vi "Noise Issues.vi"() -> ()   [LabVIEW 2013]
uses:
  <vilib>/Utility/file.llb/Read From Spreadsheet File (DBL).vi
panel:
  out "Waveform Graph":dbl[][](graph)
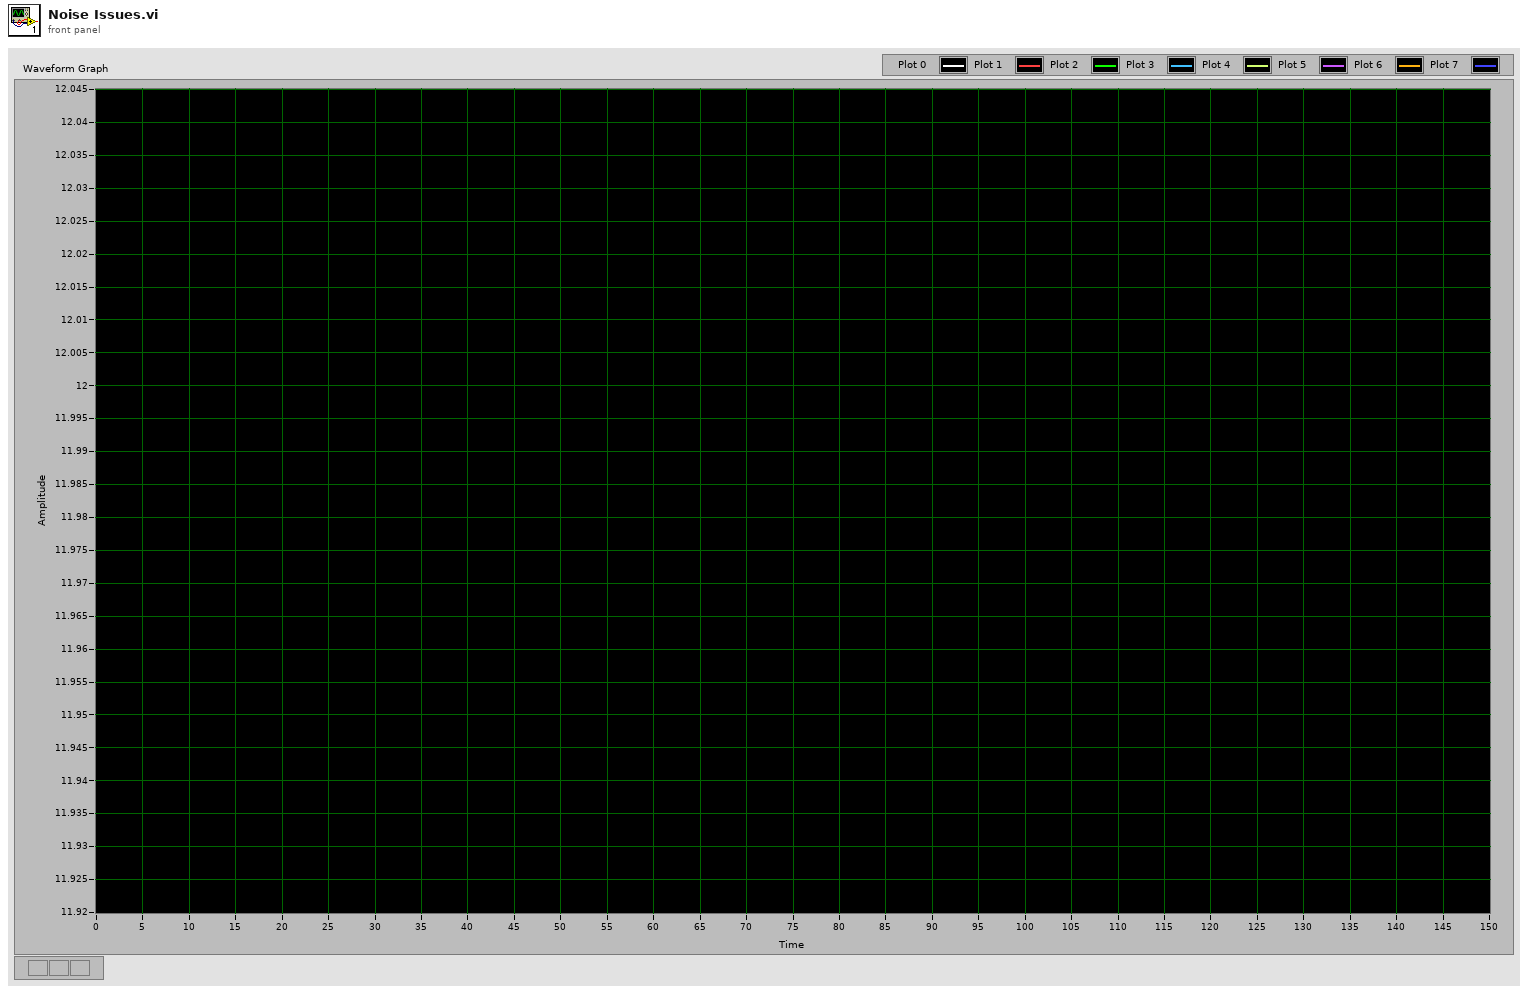
[diagram p1: front panel]
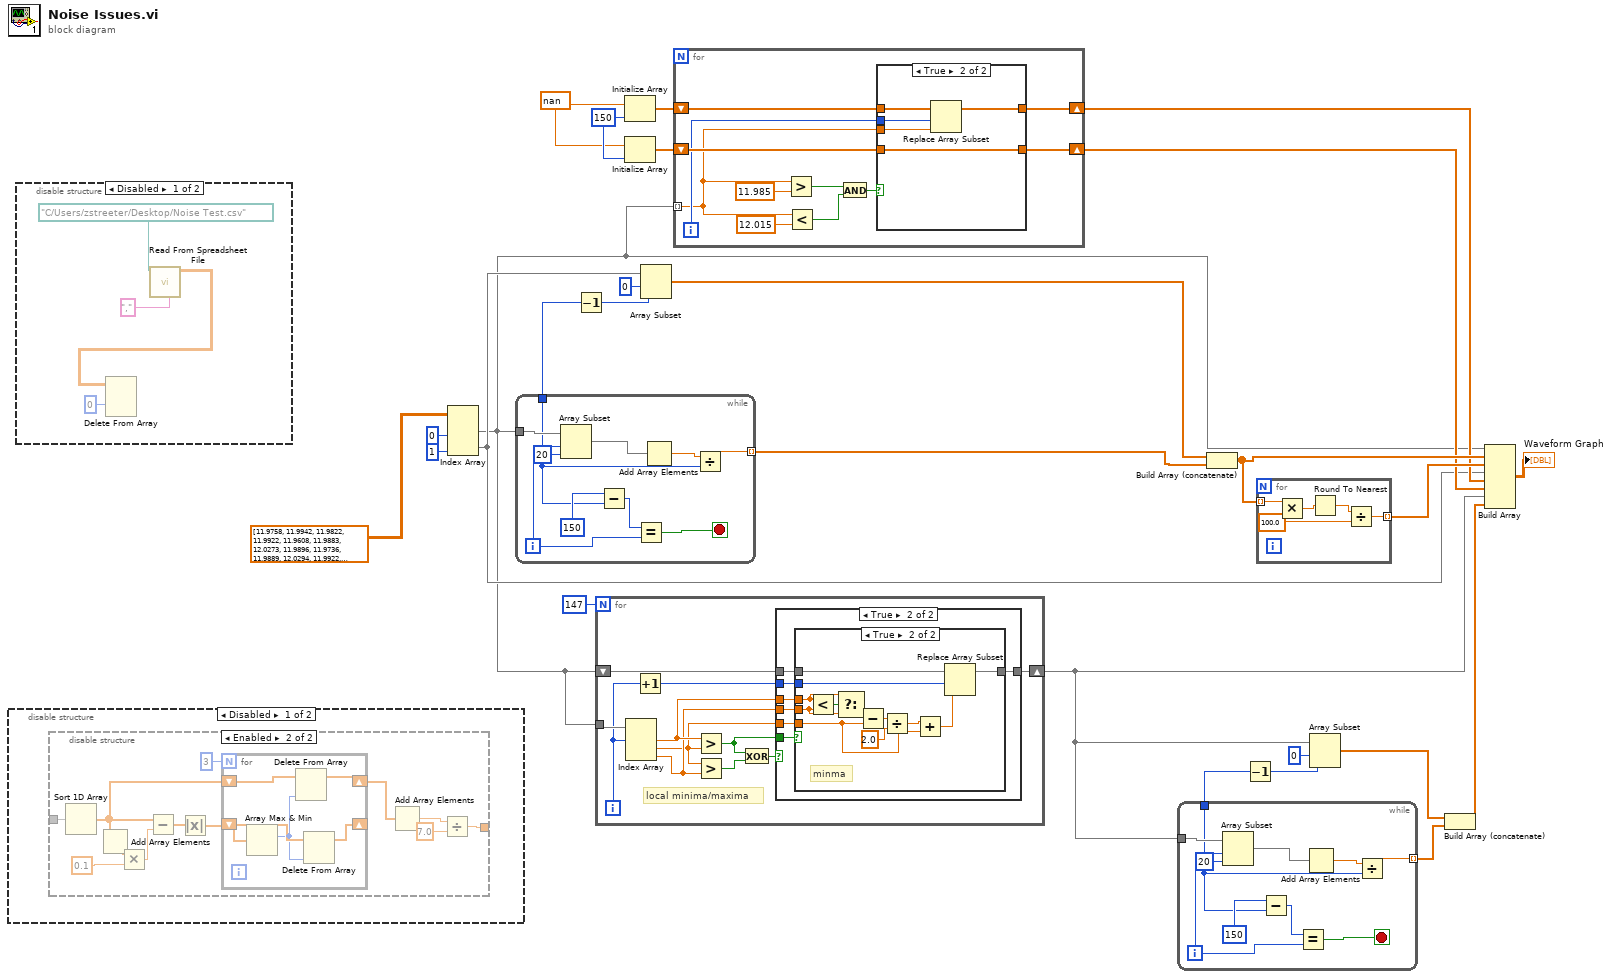
[diagram p0: block diagram]
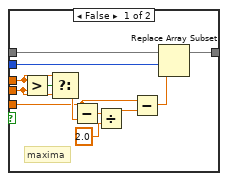
[diagram p3: hidden frame]
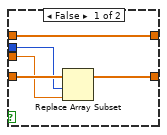
[diagram p4: hidden frame]
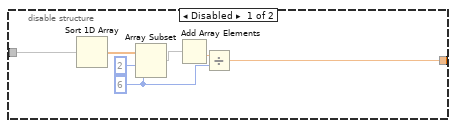
[diagram p6: hidden frame]
diagram:
  w15 = nan
  w16 = 150 ("dimension size")
  n1 = disable-structure shown="Disabled" {
    frame Disabled {
      n2 = disable-structure shown="Enabled" {
        disable-tunnel: _ -> [w34 w46]
        disable-tunnel: [w28 w38] -> _
        frame Disabled {
          w29 = 6 ("length")
          n3 = Sort 1D Array(array=w34) -> (sorted array=w33:ext[])
          n4 = Array Subset(array=w33, index=2, length=w29) -> (w31:ext[])
          n5 = Add Array Elements(numeric array=w31) -> (sum=w30:ext)
          n6 = Divide(x=w30, y=w29) -> (x/y=w28:ext)
        }
        frame Enabled {
          n7 = Sort 1D Array(array=w46) -> (sorted array=w37:ext[])
          n8 = Add Array Elements(numeric array=w37) -> (sum=w44:ext)
          n9 = Multiply(x=w44, y=0.1) -> (x*y=w43:ext)
          n10 = Subtract(x=w37, y=w43) -> (x-y=w41:ext[])
          n11 = Absolute Value(x=w41) -> (abs(x)=w36:ext[])
          n12 = for {
            N: 3 -> [_]
            shift-right: [w50] -> _
            shift-left: w36 -> [w51]
            shift-right: [w48] -> w35
            shift-left: w37 -> [w49]
            n13 = Array Max & Min(array=w51) -> (max index (indices)=w47:i32)  [unwired: 3 out]
            n14 = Delete From Array(array=w49, index=w47) -> (array with subset deleted=w48:ext[])  [unwired: 1 in, 1 out]
            n15 = Delete From Array(array=w51, index=w47) -> (array with subset deleted=w50:ext[])  [unwired: 1 in, 1 out]
          }
          n16 = Add Array Elements(numeric array=w35) -> (sum=w40:ext)
          n17 = Divide(x=w40, y=7.0) -> (x/y=w38:ext)
        }
      }
    }
    frame Enabled {
    }
  }
  n18 = disable-structure shown="Disabled" {
    frame Disabled {
      n19 = call-poly <vilib>:"Read From Spreadsheet File.vi"("delimiter (\\t)"="," ("delimiter (\\t)"), "file path (dialog if empty)"=path "C:/Users/zstreeter/Desktop/Noise Test.csv" ("new file path (Not A Path if cancelled)")) -> ("all rows"=w53:dbl[][])  [unwired: 5 in, 4 out]
      n20 = Delete From Array(array=w53, index (row)=0) -> ()  [unwired: 2 in, 2 out]
    }
    frame Enabled {
    }
  }
  n21 = Index Array(array=dbl[][] [[11.9758, 11.9942], [11.9822, 11.9922], [11.9608, 11.9883], [12.0273, 11.9896], [11.9736, 11.9889], [12.0294, 11.9922], [12.0004, 11.9922], [11.9929, 12.0003], [12.0401, 12.0018], [12.0487, 12.0031], [11.9414, 11.9997], [12.0294, 12.0044], [11.9468, 12.003], [11.8975, 11.99], [11.9811, 11.9908], [11.9543, 11.9833], [11.9715, 11.9804], [12.0358, 11.9847], [11.9511, 11.9758], [12.0101, 11.9719], [11.9736, 11.9751], [11.9779, 11.97], [12.0702, 11.9823], [11.9479, 11.9874], [11.9876, 11.988], [12.0412, 11.9967], [11.9672, 11.9963], [11.9447, 11.9871], [11.9425, 11.9863], [11.9994, 11.9852], [11.9715, 11.985], [11.9726, 11.9845], [12.0326, 11.9807], [11.9575, 11.9817], [12.0176, 11.9847], [11.9264, 11.9732], [12.0165, 11.9781], [11.9468, 11.9783], [11.9962, 11.9837], [12.0627, 11.99], [12.0519, 11.9981], [11.9565, 11.9965], [12.009, 11.9941], [11.9672, 11.9951], [11.9329, 11.9866], [12.0283, 11.9968], [11.9736, 11.9925], [11.9597, 11.9938], [12.0262, 11.9968], [12.0208, 11.9926], [12.0273, 11.9901], [11.9339, 11.9879], [12.0358, 11.9906], [11.9436, 11.9882], [11.964, 11.9913], [12.0326, 11.9918], [11.994, 11.9938], [11.9436, 11.9922], [12.0155, 11.9911], [12.0305, 11.9921], [11.9618, 11.9855], [12.0358, 11.9957], [12.0122, 11.9934], [12.0305, 12.0021], [11.9597, 12.0016], [11.9436, 11.9927], [11.9822, 11.9915], [11.9779, 11.995], [11.9189, 11.9853], [11.9479, 11.9771], [11.9597, 11.9768], [12.0122, 11.9745], [12.0208, 11.9753], [11.9146, 11.9638], [12.0069, 11.9685], [12.0616, 11.9803], [12.0573, 11.9878], [12.0273, 11.9927], [11.9779, 11.9986], [11.9232, 11.9962], [12.067, 12.0069], [11.9532, 12.001], [11.9758, 11.9965], [12.0026, 12.0053], [11.9758, 12.0022], [12.0283, 11.9988], [12.023, 11.9954], [12.0112, 11.9938], [11.9447, 11.9905], [12.0283, 12.001], [11.9726, 11.9915], [11.9833, 11.9945], [12.0176, 11.9987], [12.0305, 12.0015], [12.0358, 12.0075], [12.0358, 12.0083], [11.906, 11.9966], [12.0358, 11.999], [12.0466, 12.0092], [11.9339, 11.9998], [12.0391, 12.0065], [11.9779, 12.0059], [12.0476, 12.0089], [11.9833, 12.0042], [11.9608, 11.9967], [11.9618, 11.9893], [12.0316, 12.0018], [11.9436, 11.9926], [11.964, 11.9844], [12.0112, 11.9921], [12.067, 11.9949], [12.0112, 11.9982], [12.0058, 11.994], [12.067, 12.0024], [12.0584, 12.0121], [11.9586, 12.0118], [11.9243, 12.0011], [12.0273, 12.0095], [11.9361, 12.0067], [12.038, 12.0093], [11.9565, 11.9983], [12.0069, 11.9979], [12.0198, 11.9993], [11.9822, 11.9908], [12.024, 11.9874], [11.9522, 11.9867], [12.038, 11.9981], [11.9693, 11.9923], [12.0251, 12.0012], [11.9726, 11.9947], [11.9972, 11.9987], [12.0423, 12.0023], [12.008, 12.0011], [12.008, 12.0037], [11.9779, 11.999], [12.0208, 12.0059], [11.964, 11.9985], [12.0519, 12.0068], [11.9972, 12.004], [12.0273, 12.0095], [11.9683, 12.0066], [11.9962, 12.0019], [11.9683, 11.998], [11.9962, 11.9968], [12.0594, 12.0049], [11.9726, 12.0001], [12.0466, 12.0084], [12.0112, 12.0043], [11.8953, 11.9941], [12.0219, 11.9936]] ("array w/ subset deleted"), index (col) #1=0 ("disabled index (col)"), index (col) #2=1 ("index (col)")) -> (element #1=w8:dbl[], element #2=w9:dbl[])  [unwired: 2 in]
  n22 = while {
    tunnel: w8 -> [w64]
    tunnel: [w57] -> w19 mode=indexing
    tunnel: [w56] -> w22
    i -> [w63]
    stop <- w62 stop-if-true
    w56 = 20 ("length")
    n23 = Array Subset(array=w64, index=w63, length=w56) -> (w59:dbl[])
    n24 = Subtract(x=150, y=w56) -> (x-y=w60:i32)
    n25 = Equal?(x=w60, y=w63) -> (x = y?=w62:bool)
    n26 = Add Array Elements(numeric array=w59) -> (sum=w58:dbl)
    n27 = Divide(x=w58, y=w56) -> (x/y=w57:dbl)
  }
  n28 = Decrement(x=w22) -> (x-1=w21:i32)
  n29 = for {
    N: 147 -> [_]
    tunnel: w8 -> [w75]
    shift-right: [w71] -> w4
    shift-left: w8 -> [w73]
    i -> [w66]
    # "local minima/maxima"
    n30 = Index Array(array=w75, index #1=w66) -> (element #1=w69:dbl, element #2=w67:dbl, element #3=w68:dbl)  [unwired: 2 in]
    n31 = Increment(x=w66) -> (x+1=w65:i32)
    n32 = Greater?(x=w69, y=w67) -> (0:w70:bool)
    n33 = Greater?(x=w67, y=w68) -> (0:w74:bool)
    n34 = Exclusive Or(1:w74, 2:w70) -> (0:w72:bool)
    n35 = case shown="True" w72 {
      tunnel: w73 -> [w76 w82]
      tunnel: [w76 w78] -> w71
      tunnel: w70 -> [_ w83]
      tunnel: w69 -> [_ w81]
      tunnel: w68 -> [_ w80]
      tunnel: w67 -> [_ w79]
      tunnel: w65 -> [_ w77]
      frame False {
      }
      frame True {
        n36 = case shown="True" w83 {
          tunnel: w82 -> [w87 w103]
          tunnel: w81 -> [w94 w106]
          tunnel: w80 -> [w93 w105]
          tunnel: w79 -> [w89 w96]
          tunnel: [w86 w102] -> w78
          tunnel: w77 -> [w84 w101]
          frame False {
            # "maxima"
            n37 = Greater?(x=w94, y=w93) -> (0:w95:bool)
            n38 = Select(t=w94, s=w95, f=w93) -> (s? t:f=w92:dbl)
            n39 = Subtract(x=w89, y=w92) -> (x-y=w91:dbl)
            n40 = Divide(x=w91, y=2.0) -> (x/y=w88:dbl)
            n41 = Subtract(x=w89, y=w88) -> (x-y=w85:dbl)
            n42 = Replace Array Subset(array=w87, new element=w85, index=w84) -> (w86:dbl[])
          }
          frame True {
            # "minma"
            n43 = Less?(x=w106, y=w105) -> (x < y?=w107:bool)
            n44 = Select(t=w106, s=w107, f=w105) -> (s? t:f=w100:dbl)
            n45 = Subtract(x=w100, y=w96) -> (x-y=w99:dbl)
            n46 = Divide(x=w99, y=2.0) -> (x/y=w98:dbl)
            n47 = Add(x=w98, y=w96) -> (x+y=w97:dbl)
            n48 = Replace Array Subset(array=w103, new element=w97, index=w101) -> (w102:dbl[])
          }
        }
      }
    }
  }
  n49 = Initialize Array(w15, w16) -> (w14:dbl[])
  n50 = Initialize Array(w15, w16) -> (w13:dbl[])
  n51 = Array Subset(array=w9, index=0, length=w21) -> (w24:dbl[])
  n52 = for {
    shift-right: [w116] -> w11
    shift-left: w14 -> [w118]
    shift-right: [w113] -> w12
    shift-left: w13 -> [w117]
    tunnel: w8 -> [w114] mode=indexing
    i -> [w115]
    n53 = Greater?(x=w114, y=11.985) -> (0:w111:bool)
    n54 = Less?(x=w114, y=12.015) -> (x < y?=w110:bool)
    n55 = And(x=w111, y=w110) -> (x .and. y?=w112:bool)
    n56 = case shown="True" w112 {
      tunnel: w118 -> [w119 w128]
      tunnel: w117 -> [w123 w124]
      tunnel: [w119 w127] -> w116
      tunnel: w115 -> [w121 w126]
      tunnel: w114 -> [w120 w125]
      tunnel: [w122 w124] -> w113
      frame False {
        n57 = Replace Array Subset(array=w123, new element=w120, index=w121) -> (w122:dbl[])
      }
      frame True {
        n58 = Replace Array Subset(array=w128, new element=w125, index=w126) -> (w127:dbl[])
      }
    }
  }
  n59 = while {
    tunnel: w4 -> [w137]
    tunnel: [w130] -> w2 mode=indexing
    tunnel: [w129] -> w5
    i -> [w136]
    stop <- w135 stop-if-true
    w129 = 20 ("length")
    n60 = Array Subset(array=w137, index=w136, length=w129) -> (w132:dbl[])
    n61 = Subtract(x=150, y=w129) -> (x-y=w133:i32)
    n62 = Equal?(x=w133, y=w136) -> (x = y?=w135:bool)
    n63 = Add Array Elements(numeric array=w132) -> (sum=w131:dbl)
    n64 = Divide(x=w131, y=w129) -> (x/y=w130:dbl)
  }
  n65 = Build Array (concatenate)(w24, w19) -> (w18:dbl[])
  n66 = Decrement(x=w5) -> (x-1=w7:i32)
  n67 = for {
    tunnel: w18 -> [w142] mode=indexing
    tunnel: [w138] -> w17 mode=indexing
    w141 = 100.0
    n68 = Multiply(x=w142, y=w141) -> (x*y=w140:dbl)
    n69 = Round To Nearest(number=w140) -> (nearest integer value=w139:dbl)
    n70 = Divide(x=w139, y=w141) -> (x/y=w138:dbl)
  }
  n71 = Array Subset(array=w4, index=0, length=w7) -> (w3:dbl[])
  n72 = Build Array (concatenate)(w3, w2) -> (w1:dbl[])
  n73 = Build Array(w8, w18, w17, w9, w11, w12, w4, w1) -> (→"Waveform Graph":dbl[][])
